vi "Api Version Check.vi"(8 "error in (no error)":errorcluster, 11 "version":u32) -> (0 "error out":errorcluster)   [LabVIEW 2026, in "MrcLib.lvlib"]
doc: "Verify that the version of the API you intend to use is compatible with the libraries on the robot controller."
uses:
  MrcLib.lvlib
panel:
  out "Version Pass":bool
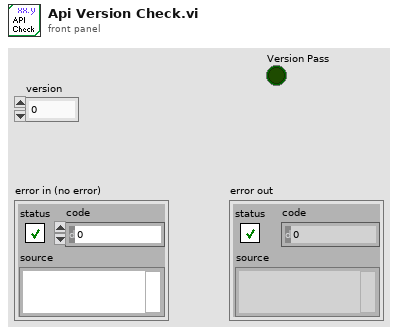
[diagram p1: front panel]
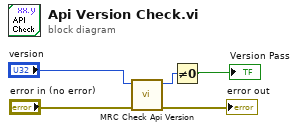
[diagram p0: block diagram]
diagram:
  n1 = call "MRC Check Api Version.vi"("error in (no error)"="error in (no error)", "version"="version") -> ("error out"=→"error out":errorcluster, "function return"=w3:u8)  [unwired: 8 in]
  n2 = Not Equal To 0?(x=w3) -> (x != 0?=→"Version Pass":bool)
